vi "Close.vi"(8 "error in (no error)":errorcluster, 10 "Msg in":T1, 11 "Hexapod":refnum<class "Tapedrive_ESP301.lvclass">) -> (0 "error out":errorcluster, 1 "new command":string, 2 "Msg out":T1, 3 "Hexapod out":refnum<class "Tapedrive_ESP301.lvclass">)   [LabVIEW 2013, in "Tapedrive_ESP301.lvclass"]
uses:
  Tapedrive_ESP301.lvclass
  BaseDriver/BaseDriver.lvclass
  BaseDriver/DriverMsg.ctl
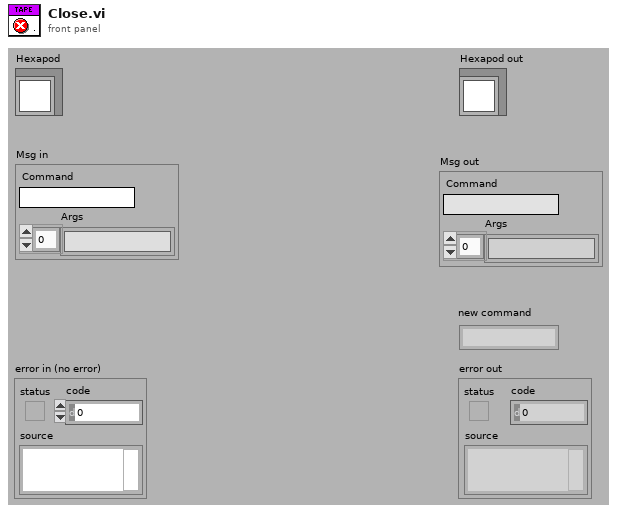
[diagram p1: front panel]
types:
  T1 = typedef "DriverMsg.ctl" = cluster{"Command":string, "Args":string[]}
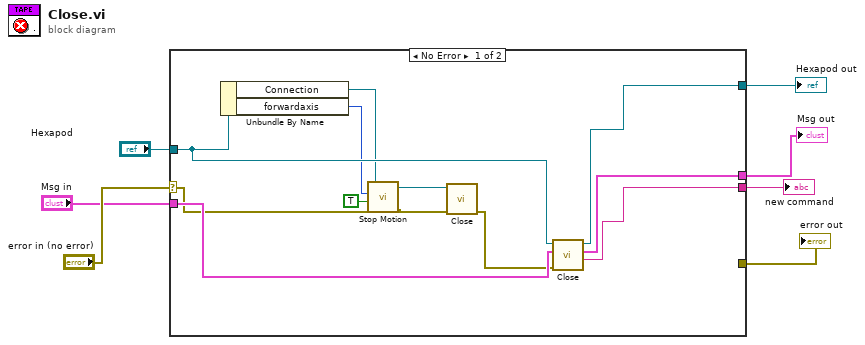
[diagram p0: block diagram]
diagram:
  n1 = case shown="No Error" "error in (no error)" {
    selector: "error in (no error)" -> [w11 w22]
    tunnel: [_ w22] -> w7
    tunnel: "Hexapod" -> [w19 w20]
    tunnel: "Msg in" -> [w18 w21]
    tunnel: [w17 w20] -> w3
    tunnel: [w16 w21] -> w2
    tunnel: [w15 _] -> w1
    frame No Error {
      n2 = Unbundle By Name(w19) -> ("Connection"=w12:refnum<visa-resource-name>, "forwardaxis"=w8:i16)
      n3 = call <instrlib>:"Stop Motion.vi"("error in (no error)"=w11, "Stop all axes (F)"=TRUE, "Axis (1)"=w8, "VISA resource name"=w12) -> ("error out"=w10:errorcluster, "VISA resource name out"=w13:refnum<visa-resource-name>)  [unwired: 2 in]
      n4 = call <instrlib>:"Close.vi"("error in (no error)"=w10, "VISA resource name"=w13) -> ("error out"=w14:errorcluster)  [unwired: 9 in]
      n5 = call-parent <instrlib>:"Close.vi"("error in (no error)"=w14, "Msg in"=w18, "BaseDriver in"=w19) -> ("new command"=w15:string, "Msg out"=w16:T1, "BaseDriver out"=w17:refnum<class "Tapedrive_ESP301.lvclass">)  [unwired: 5 in, 1 out]
    }
    frame Error {
    }
  }
  "error out" <- w7
  "new command" <- w1
  "Msg out" <- w2
  "Hexapod out" <- w3
